vi "Get Zero Offset Mode.vi"(8 "error in (no error)":errorcluster, 11 "VISA resource name":refnum<visa-resource-name>) -> (0 "error out":errorcluster, 1 "Reference Value":dbl format="%.4f", 2 "Zero Offset Mode":u16, 3 "VISA resource name out":refnum<visa-resource-name>, 4 "Reference Value Units":i32)   [LabVIEW 2013, in "Fluke 5XXX Series Multicalibrators.lvlib"]
doc: "This VI returns the zero offset for the pressure module or capacitance measurement using the oscilloscope option.\n\nNote:\n\nThis VI is available only for instrument models 5500A and 5520A with oscilloscope option SC600 (SC1100) or option 700P (pressure modules)."
uses:
  Fluke 5XXX Series Multicalibrators.lvlib
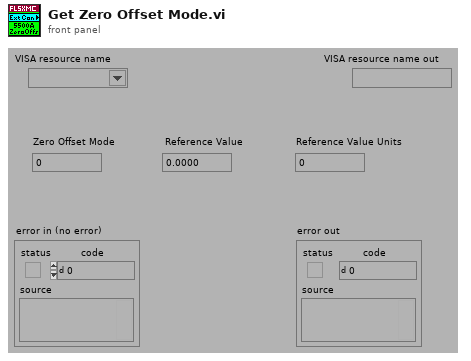
[diagram p1: front panel]
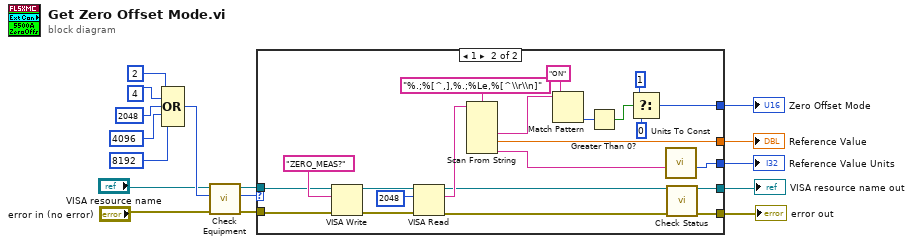
[diagram p0: block diagram]
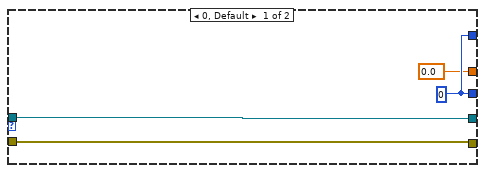
[diagram p2: hidden frame]
diagram:
  n1 = Compound Arithmetic op=OR(2 ("Numeric"), 4 ("Numeric"), 2048 ("Numeric"), 4096 ("Numeric"), 8192 ("Numeric")) -> (w8:i32)
  n2 = call "Check Equipment.vi"("error in (no error)"="error in (no error)", "Bit Mask"=w8, "VISA resource name"="VISA resource name") -> ("error out"=w16:errorcluster, "Present?"=w15:u32, "VISA resource name out"=w14:refnum<visa-resource-name>)  [unwired: 6 in]
  n3 = case shown="1" w15 {
    tunnel: [w20 w36] -> w5
    tunnel: [w19 w35] -> w4
    tunnel: w16 -> [w20 w38]
    tunnel: w14 -> [w19 w37]
    tunnel: [w18 w23] -> w3
    tunnel: [w18 w22] -> w1
    tunnel: [0.0 w21] -> w2
    frame 0, Default {
      w18 = 0
    }
    frame 1 {
      n4 = VISA Write(VISA resource name=w37, write buffer="ZERO_MEAS?", error in (no error)=w38) -> (VISA resource name out=w41:refnum<visa-resource-name>, error out=w40:errorcluster)  [unwired: 1 out]
      n5 = VISA Read(VISA resource name=w41, byte count=u32 2048 ("byte count (0)"), error in (no error)=w40) -> (VISA resource name out=w31:refnum<visa-resource-name>, read buffer=w33:string, error out=w32:errorcluster)  [unwired: 1 out]
      n6 = Scan From String(format string="%.;%[^,],%.;%Le,%[^\\r\\n]", input string=w33) -> (output 1=w25:string, output 2=w21:dbl, output 3=w24:string)  [unwired: 5 in, 3 out]
      n7 = Match Pattern(string=w25, regular expression="ON") -> (offset past match=w29:i32)  [unwired: 1 in, 3 out]
      n8 = Greater Than 0?(x=w29) -> (x > 0?=w26:bool)
      n9 = Select(t=u16 1 ("f"), s=w26, f=u16 0) -> (s? t:f=w22:u16)
      n10 = call "Units To Const.vi"("Units"=w24) -> ("Const"=w23:i32)  [unwired: 10 in]
      n11 = call "Check Status.vi"("VISA resource name"=w31, "error in (no error)"=w32) -> ("VISA resource name out"=w35:refnum<visa-resource-name>, "error out"=w36:errorcluster)  [unwired: 12 in]
    }
  }
  "Zero Offset Mode" <- w1
  "Reference Value" <- w2
  "Reference Value Units" <- w3
  "VISA resource name out" <- w4
  "error out" <- w5
